vi "Launch as Nested.vi"(6 "Client":refnum<k5>, 8 "error in (no error)":errorcluster, 9 "Port":u16, 10 "Address":string, 11 "Parent in":refnum<class "Module.lvclass">) -> (0 "error out":errorcluster, 2 "MessageQ":refnum<class "MessageQ.lvclass">, 3 "Parent":refnum<class "Module.lvclass">)   [LabVIEW 2020, in "Volatus.lvlib" / "Messaging Server Client.lvclass"]
uses:
  Messaging Server Client.lvclass
  Messaging Server Client.lvclass/Messaging Server Client.ctl
  Module/Module.lvclass
  VolatusConfig/VolatusConfigElement/VolatusConfigElement.lvclass
  Volatus.lvlib
  C:/dev/lv20CE/relink/lv-volatus/Volatus/Module/Module.lvclass
  C:/dev/lv20CE/relink/lv-volatus/Volatus/Messaging Client/Messaging Server Client.lvclass
  MessageQ/MessageQ.lvclass
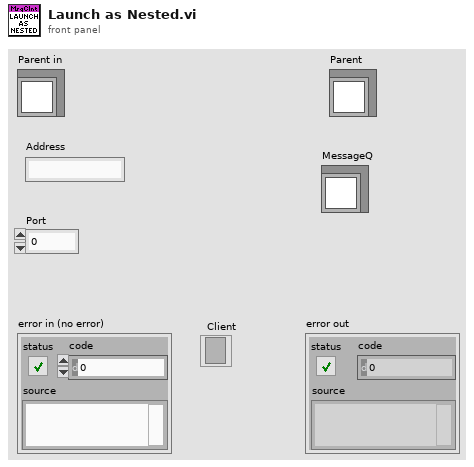
[diagram p1: front panel]
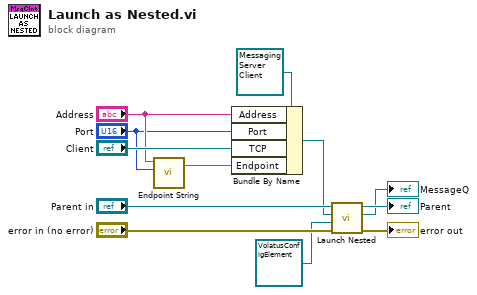
[diagram p0: block diagram]
diagram:
  n1 = call "Endpoint String.vi"("Port"="Port", "Address"="Address") -> ("Endpoint"=w1:string)  [unwired: 3 in]
  n2 = Bundle By Name(cluster=refnum<class "Messaging Server Client.lvclass"> refnum ("Volatus:Messaging Client.lvclass"), "Address"="Address", "Port"="Port", "TCP"="Client", "Endpoint"=w1) -> (w7:refnum<class "Messaging Server Client.lvclass">)
  n3 = call "Launch Nested.vi"("error in (no error)"="error in (no error)", "Config Element"=refnum<class "VolatusConfigElement.lvclass"> refnum, "Nested Module"=w7, "Parent in"="Parent in") -> ("error out"=→"error out":errorcluster, "MessageQ"=→"MessageQ":refnum<class "MessageQ.lvclass">, "Parent out"=→"Parent":refnum<class "Module.lvclass">)  [unwired: 5 in]
